vi "参数配置表.vi"() -> ()   [LabVIEW 2016, in "数据传输系统.lvlib"]
uses:
  <vilib>/Utility/miscctls.llb/LVPointTypeDef.ctl
  <vilib>/Utility/config.llb/NI_LVConfig.lvlib
  <vilib>/ptbypt/NI_PtbyPt.lvlib
panel:
  in  "加密传输":bool
  in  "数据库类型":enum16{"Access", "SQLite"}(ring)
  in  "应用环境":enum16{"STD", "GB212"}(ring)
  in  "屏蔽维护数据":bool
  in  "数据发送延时时间/s":i32
  in  "判断数据反馈":enum16{"非严格判断", "严格判断", "不判断"}(ring)
  in  "仪器参数发送":bool
  in  "地表水/污染源":bool
  in  "间隔时间/分钟":i32
  in  "数据发送通道":enum16{"TCP", "VISA"}(ring)
  in  "数据发送协议":enum16{"2005-212协议", "2017-212协议"}(ring)=enum."2017-212协议"
  in  "数据触发上传方式":enum16{"出数即刻发送", "间隔时间发送", "整点发送"}(ring)
  in  "数据组合发送":bool
  in  "日志、参数发送":bool
  in  "2011发送":bool
  in  "返回":bool
  out "配置表格":string[][](table)
  in  "参数数值":T1={"CODMn"=TRUE, "CODCr"=TRUE, "DO"=TRUE, "铜"=TRUE, "PH"=TRUE, "氨氮"=TRUE, "比电导率"=TRUE, "水温"=TRUE, "COD"=TRUE, "浊度"=TRUE, "总氮"=TRUE, "总磷"=TRUE, "叶绿素a"=TRUE, "藻密度"=TRUE, "水位"=TRUE, "流速"=TRUE, "瞬时流量"=TRUE, "累积流量"=TRUE, "亚硝氮"=TRUE, "硫化物"=TRUE, "ORP"=TRUE, "铅"=TRUE, "镉"=TRUE, "锌"=TRUE, "镍"=TRUE, "锰"=TRUE, "汞"=TRUE, "气温"=TRUE, "气压"=TRUE, "风速"=TRUE, "风向"=TRUE, "盐度"=TRUE, "磷酸盐"=TRUE, "硝氮"=TRUE, "氟化物"=TRUE}
  # "因子编码，单位配置，上传功能码，小时、质控数据上传触发方式"
  # "参数配置"
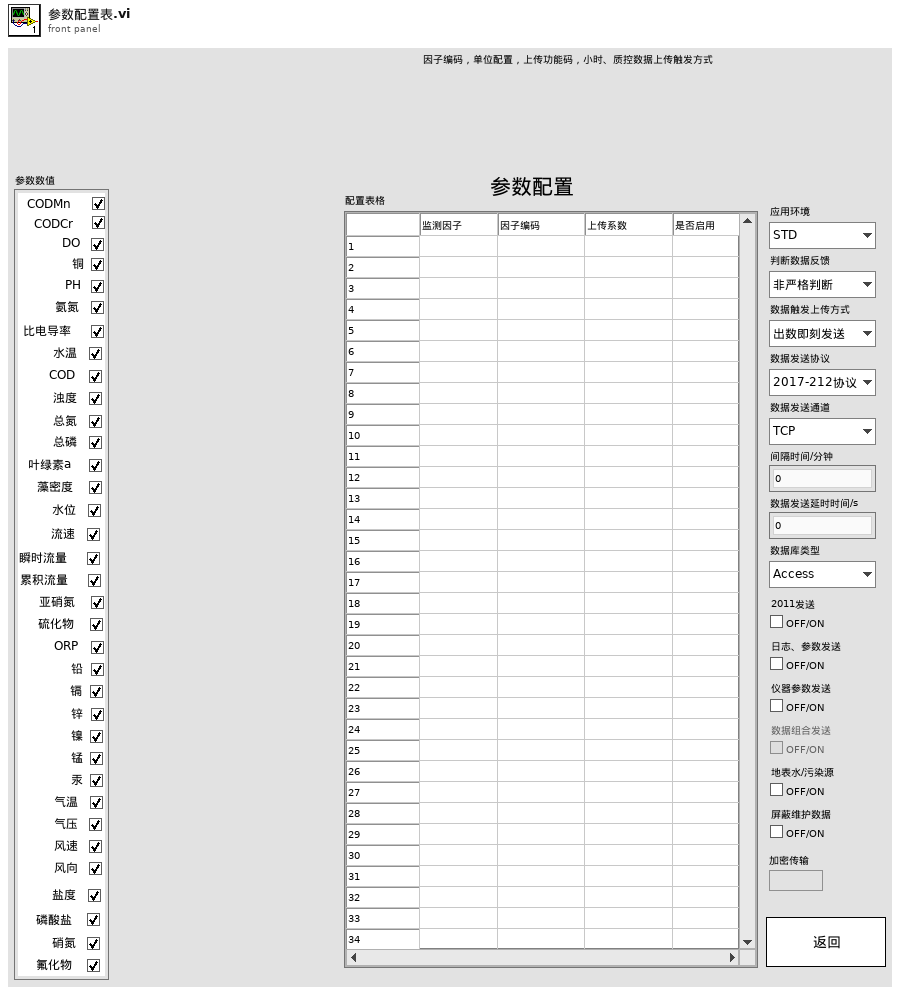
[diagram p1: front panel]
types:
  T1 = cluster{"CODMn":bool, "CODCr":bool, "DO":bool, "铜":bool, "PH":bool, "氨氮":bool, "比电导率":bool, "水温":bool, "COD":bool, "浊度":bool, "总氮":bool, "总磷":bool, "叶绿素a":bool, "藻密度":bool, "水位":bool, "流速":bool, "瞬时流量":bool, "累积流量":bool, "亚硝氮":bool, "硫化物":bool, "ORP":bool, "铅":bool, "镉":bool, "锌":bool, "镍":bool, "锰":bool, "汞":bool, "气温":bool, "气压":bool, "风速":bool, "风向":bool, "盐度":bool, "磷酸盐":bool, "硝氮":bool, "氟化物":bool}
  T2 = typedef "LVPointTypeDef.ctl" = cluster{"Horizontal":i16, "Vertical":i16}
  T3 = typedef "NI_LVConfig.lvlib/Config Data RefNum.ctl" = refnum<k1>
  T4 = cluster{"[0]":string, "[1]":string, "[2]":string, "[3]":string, "[4]":string, "[5]":string, "[6]":string, "[7]":string, "[8]":string, "[9]":string, "[10]":string, "[11]":string, "[12]":string, "[13]":string, "[14]":string, "[15]":string, "[16]":string, "[17]":string, "[18]":string, "[19]":string, "[20]":string, "[21]":string, "[22]":string, "[23]":string, "[24]":string, "[25]":string, "[26]":string, "[27]":string, "[28]":string, "[29]":string, "[30]":string, "[31]":string, "[32]":string, "[33]":string, "[34]":string}
  T5 = enum8{"Enabled", "Disabled", "Disabled and Grayed Out"}
  T6 = typedef "LVRowAndColumnTypeDef.ctl" = cluster{"Row":i32, "Column":i32}
  T7 = cluster{"[0]":string, "[1]":string, "[2]":string, "[3]":string, "[4]":string, "[5]":string, "[6]":string}
  T8 = cluster{"[0]":string, "[1]":string, "[2]":string, "[3]":string, "[4]":string, "[5]":string, "[6]":string, "[7]":string, "[8]":string, "[9]":string, "[10]":string, "[11]":string, "[12]":string}
  T9 = cluster{"[0]":string, "[1]":string, "[2]":string, "[3]":string, "[4]":string, "[5]":string, "[6]":string, "[7]":string, "[8]":string, "[9]":string, "[10]":string, "[11]":string, "[12]":string, "[13]":string}
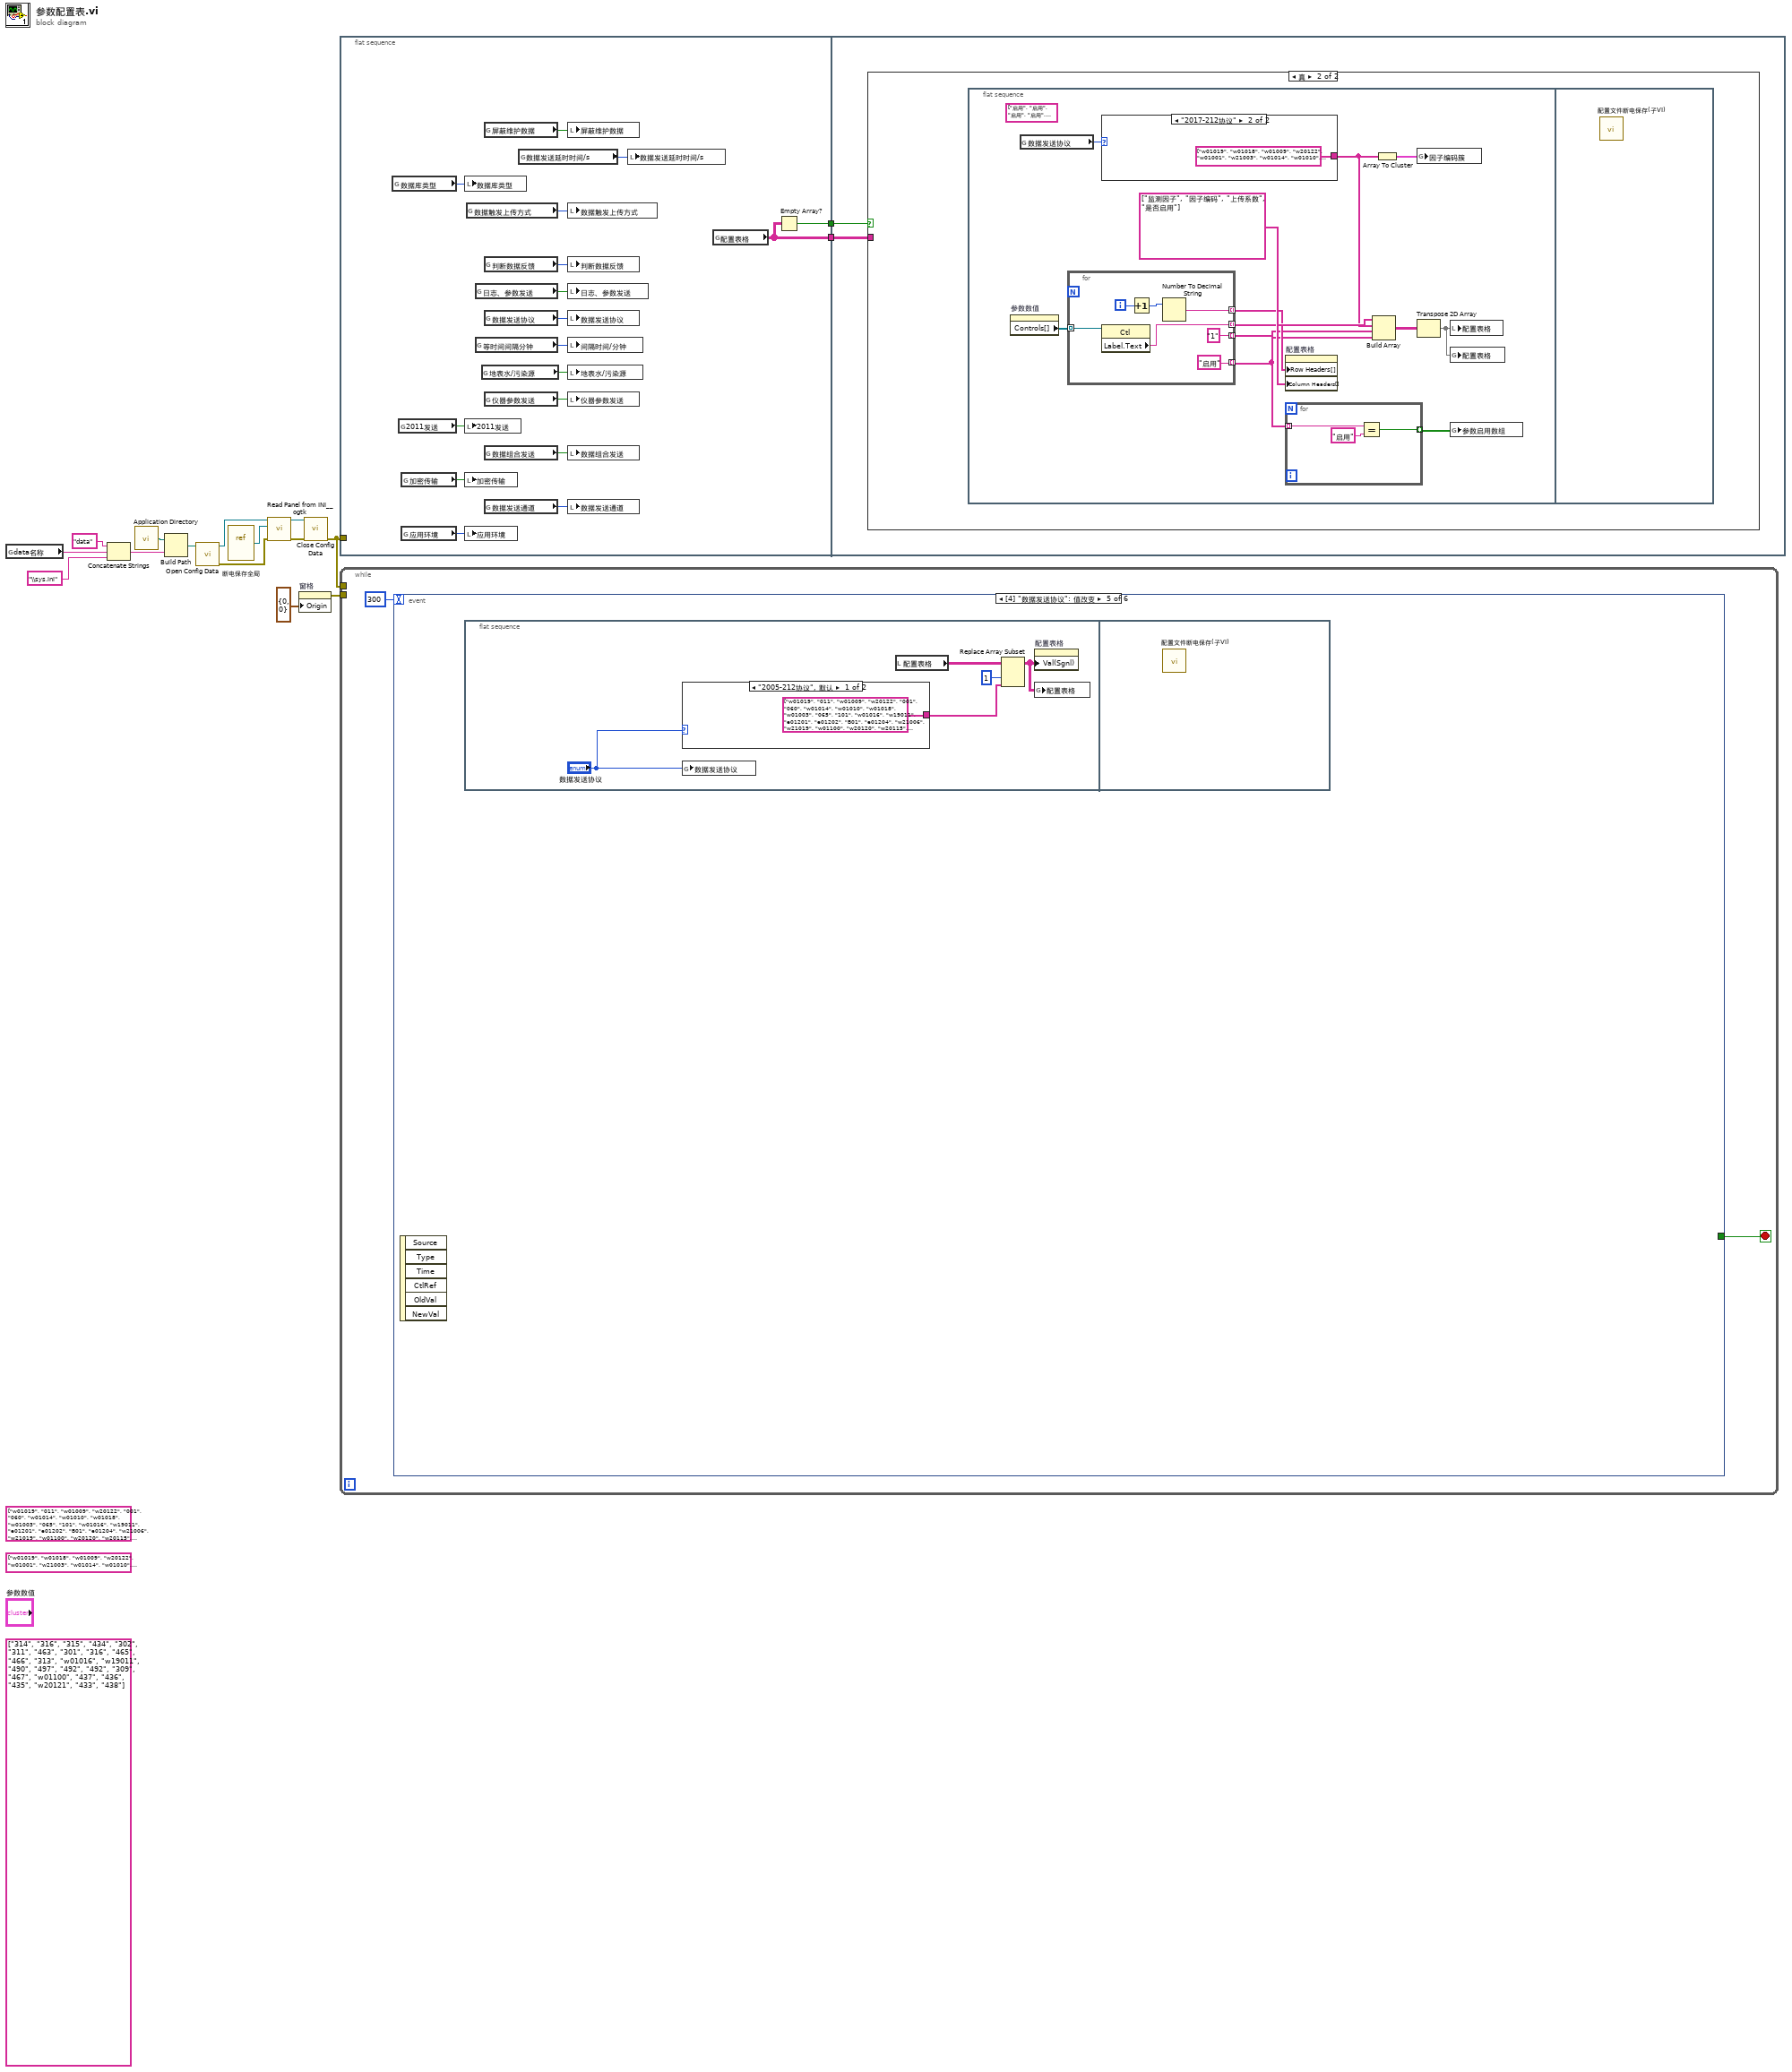
[diagram p0: block diagram]
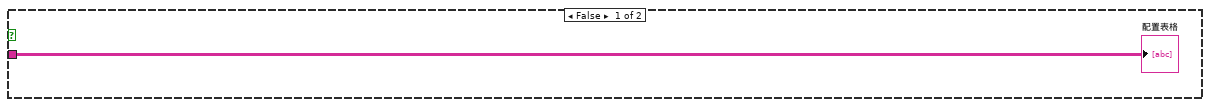
[diagram p2: hidden frame]
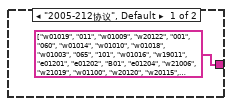
[diagram p3: hidden frame]
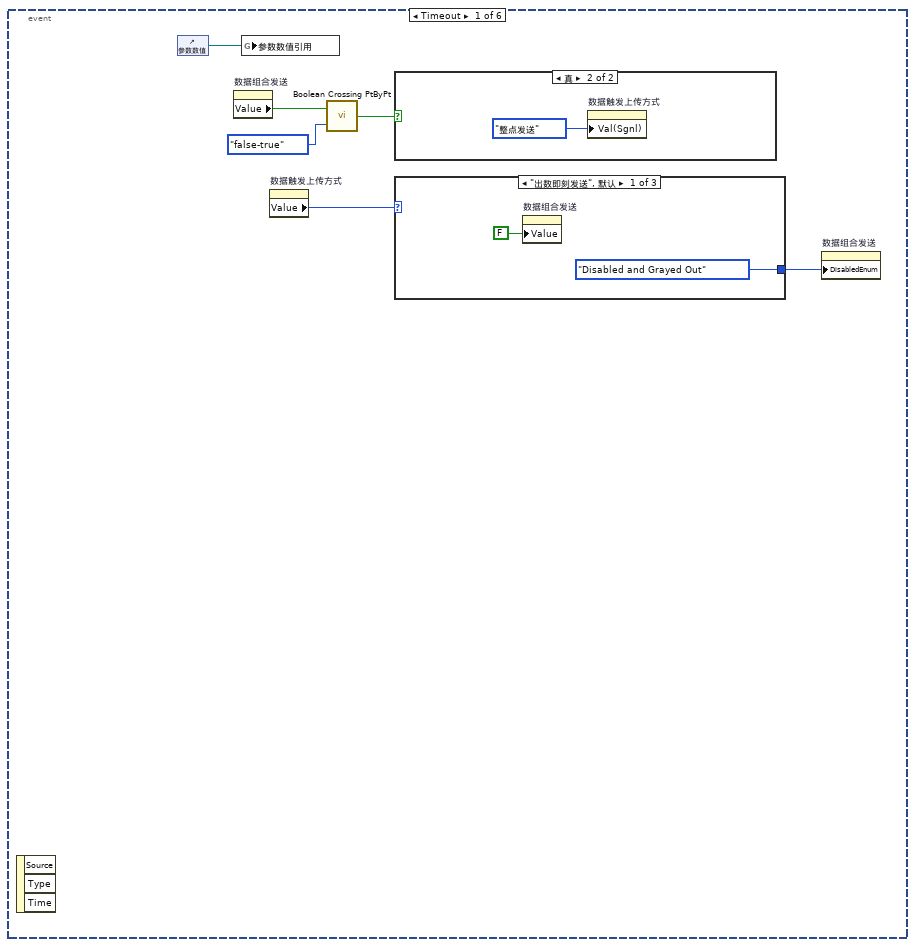
[diagram p4: hidden frame]
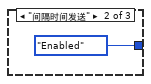
[diagram p6: hidden frame]
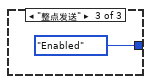
[diagram p7: hidden frame]
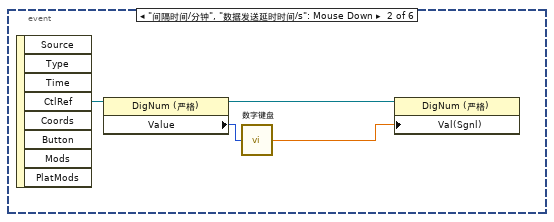
[diagram p8: hidden frame]
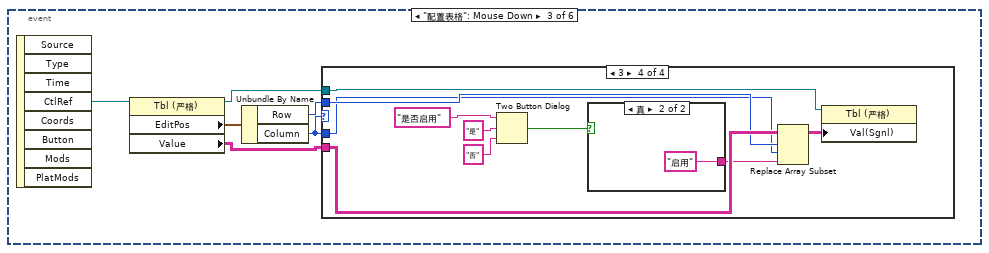
[diagram p9: hidden frame]
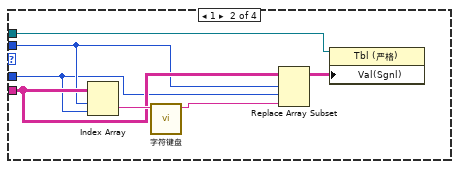
[diagram p11: hidden frame]
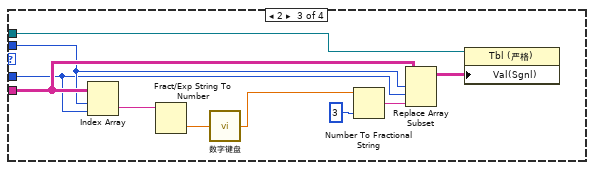
[diagram p12: hidden frame]
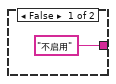
[diagram p13: hidden frame]
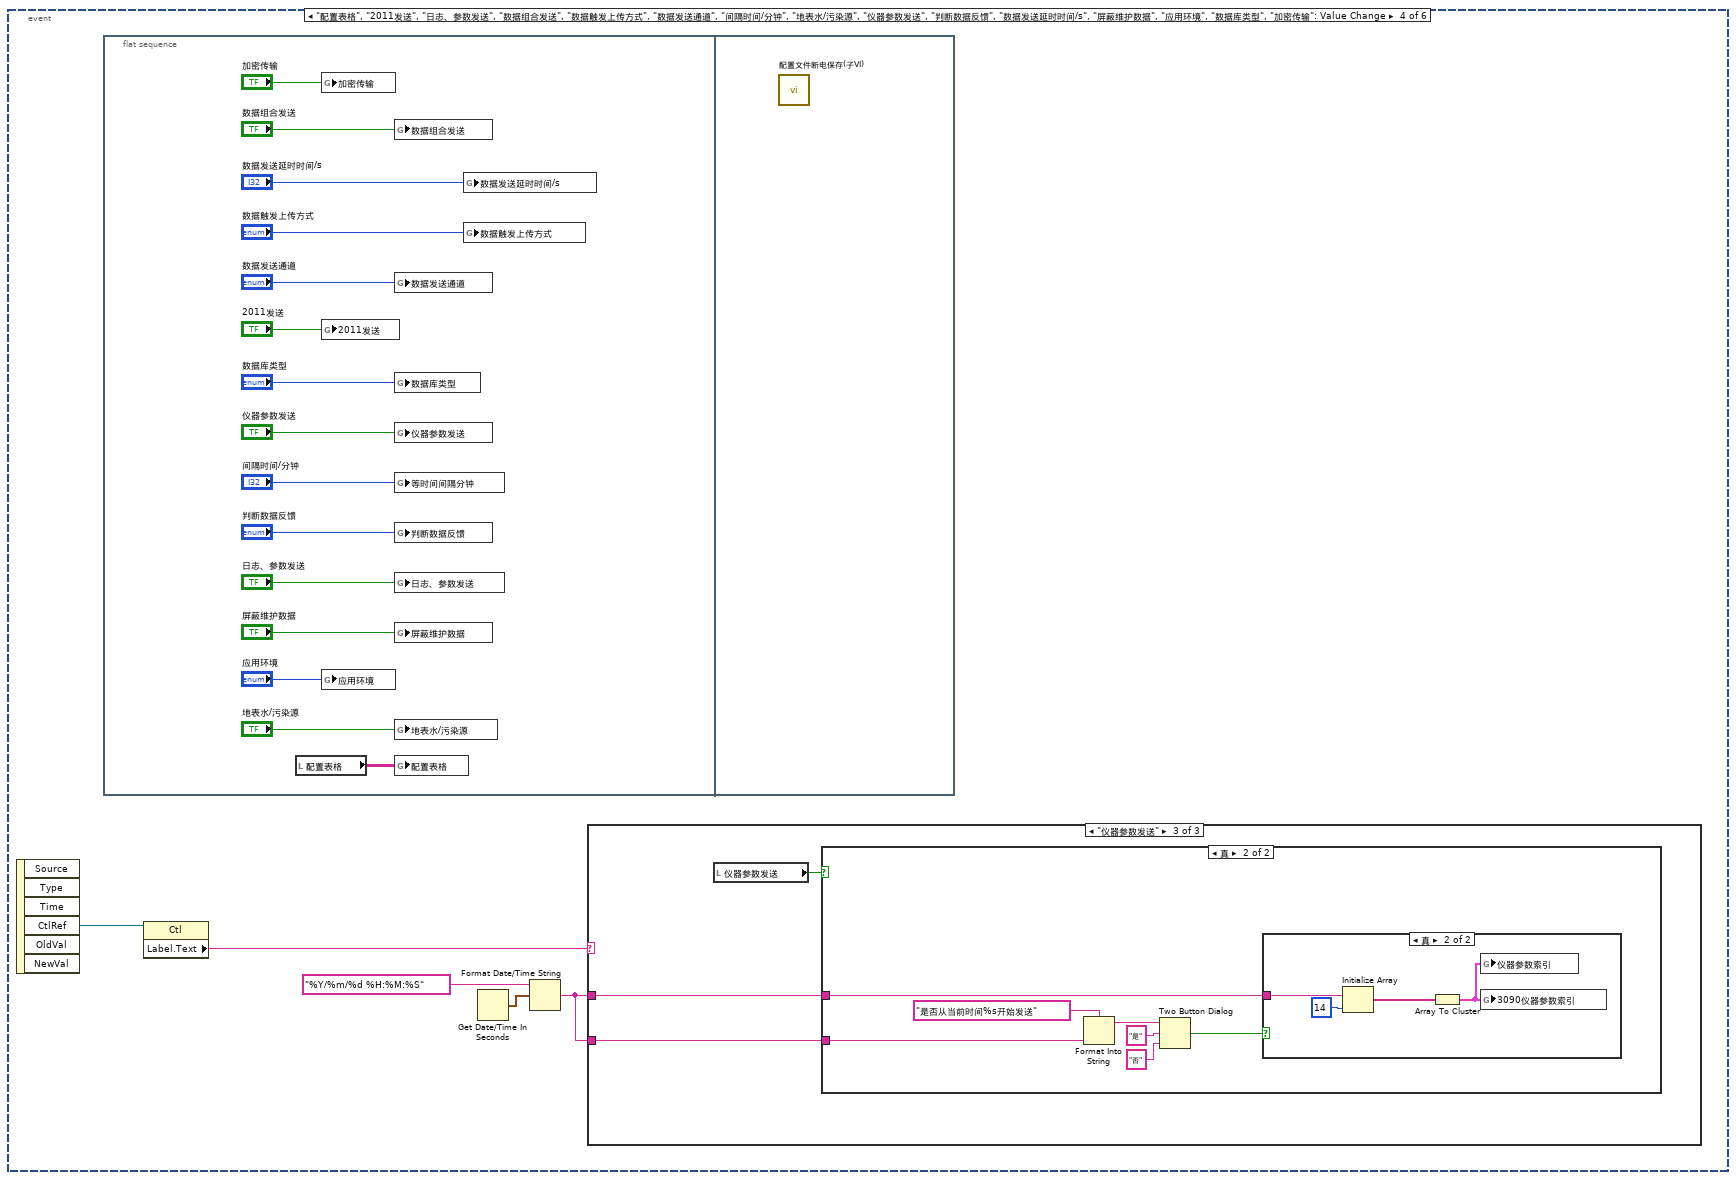
[diagram p14: hidden frame]
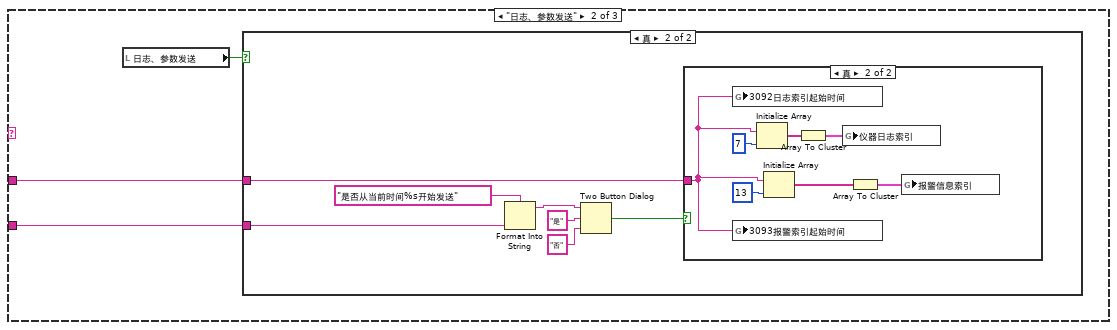
[diagram p16: hidden frame]
diagram:
  (unwired) string[] ["w01019", "011", "w01009", "w20122", "001", "060", "w01014", "w01010", "w01018", "w01003", "065", "101", "w01016", "w19011", "e01201", "e01202", "B01", "e01204", "w21006", "w21019", "w01100", "w20120", "w20115", "w20123", "w20121", "w20124", "w20111", "a01001", "a01006", "a01007", "a01008", "w01002", "w21015", "w21007", "w21017"]
  (unwired) string[] ["w01019", "w01018", "w01009", "w20122", "w01001", "w21003", "w01014", "w01010", "w01018", "w01003", "w21001", "w21011", "w01016", "w19011", "e01201", "e01202", "e01203", "e01204", "w21006", "w21019", "w01100", "w20120", "w20115", "w20123", "w20121", "w20124", "w20111", "a01001", "a01006", "a01007", "a01008", "w01002", "w21015", "w21007", "w21017"]
  (unwired) string[] ["314", "316", "315", "434", "302", "311", "463", "301", "316", "465", "466", "313", "w01016", "w19011", "490", "497", "492", "492", "309", "467", "w01100", "437", "436", "435", "w20121", "433", "438"]
  n1 = global read "断电保存全局.vi" "data名称"() -> (w3:string)
  n2 = Concatenate Strings("data" ("名称或相对路径"), w3, "\\sys.ini" ("名称或相对路径")) -> (w1:string)
  n3 = call <vilib>:"Application Directory.vi"() -> ("Application Directory"=w12:path)
  n4 = Build Path(base path=w12, name or relative path=w1) -> (appended path=w11:path)
  n5 = call <vilib>:"Open Config Data.vi"("configuration file path"=w11) -> ("error out"=w16:errorcluster, "refnum"=w15:T3)  [unwired: 8 in, 1 out]
  n6 = vi-ref "断电保存全局.vi"() -> (w14:refnum<vi>)
  n7 = call <userlib>:"Read Panel from INI__ogtk.vi"("error in (no error)"=w16, "VI ref"=w14, "refnum"=w15) -> ("error out"=w10:errorcluster, "refnum out"=w13:T3)  [unwired: 7 in]
  n8 = property on="窗格" class="Pane"("Origin"=T2 {"Horizontal"=0, "Vertical"=0} ("原点")) -> (error out=w8:errorcluster)  [unwired: 2 in, 1 out]
  n9 = call <vilib>:"Close Config Data.vi"("error in (no error)"=w10, "refnum"=w13) -> ("error out"=w9:errorcluster)  [unwired: 8 in, 1 out]
  n10 = flat-sequence {
    tunnel: w9 -> [_]
    tunnel: [w26] -> w6
    tunnel: [w25] -> w5
    tunnel: w6 -> [w35]
    tunnel: w5 -> [w34]
    frame #0 {
      n11 = global read "断电保存全局.vi" "数据库类型"() -> (w18:enum16{"Access", "SQLite"})
      n12 = global read "断电保存全局.vi" "2011发送"() -> (w33:bool)
      n13 = global read "断电保存全局.vi" "加密传输"() -> (w17:bool)
      n14 = global read "断电保存全局.vi" "应用环境"() -> (w19:enum16{"STD", "GB212"})
      n15 = local write "数据库类型"(w18) -> ()
      n16 = local write "2011发送"(w33) -> ()
      n17 = local write "加密传输"(w17) -> ()
      n18 = local write "应用环境"(w19) -> ()
      n19 = global read "断电保存全局.vi" "数据触发上传方式"() -> (w29:enum16{"出数即刻发送", "间隔时间发送", "整点发送"})
      n20 = global read "断电保存全局.vi" "日志、参数发送"() -> (w31:bool)
      n21 = global read "断电保存全局.vi" "等时间间隔分钟"() -> (w24:i32)
      n22 = global read "断电保存全局.vi" "地表水/污染源"() -> (w23:bool)
      n23 = global read "断电保存全局.vi" "屏蔽维护数据"() -> (w20:bool)
      n24 = global read "断电保存全局.vi" "判断数据反馈"() -> (w32:enum16{"非严格判断", "严格判断", "不判断"})
      n25 = global read "断电保存全局.vi" "数据发送协议"() -> (w27:enum16{"2005-212协议", "2017-212协议"})
      n26 = global read "断电保存全局.vi" "仪器参数发送"() -> (w22:bool)
      n27 = global read "断电保存全局.vi" "数据组合发送"() -> (w30:bool)
      n28 = global read "断电保存全局.vi" "数据发送通道"() -> (w28:enum16{"TCP", "VISA"})
      n29 = global read "断电保存全局.vi" "数据发送延时时间/s"() -> (w21:i32)
      n30 = local write "屏蔽维护数据"(w20) -> ()
      n31 = local write "数据触发上传方式"(w29) -> ()
      n32 = local write "判断数据反馈"(w32) -> ()
      n33 = local write "日志、参数发送"(w31) -> ()
      n34 = local write "数据发送协议"(w27) -> ()
      n35 = local write "间隔时间/分钟"(w24) -> ()
      n36 = local write "地表水/污染源"(w23) -> ()
      n37 = local write "仪器参数发送"(w22) -> ()
      n38 = local write "数据组合发送"(w30) -> ()
      n39 = local write "数据发送通道"(w28) -> ()
      n40 = local write "数据发送延时时间/s"(w21) -> ()
      n41 = global read "断电保存全局.vi" "配置表格"() -> (w25:string[][])
      n42 = Empty Array?(array=w25) -> (empty?=w26:bool)
    }
    frame #1 {
      n43 = case shown="真" w35 {
        tunnel: w34 -> [w36 _]
        frame False {
          "配置表格" <- w36
        }
        frame True {
          n44 = flat-sequence {
            frame #0 {
              (unwired) string[] ["启用", "启用", "启用", "启用", "启用", "启用", "启用", "启用", "启用", "启用", "启用", "启用", "启用", "启用", "启用", "启用", "启用", "启用", "启用", "启用", "启用", "启用", "启用", "启用", "启用", "启用", "启用"]
              n45 = property on="参数数值" class="Clust (严格)"() -> ("Controls[]"=w44:refnum<vi>[])  [unwired: 2 in, 2 out]
              n46 = global read "断电保存全局.vi" "数据发送协议"() -> (w42:enum16{"2005-212协议", "2017-212协议"})
              n47 = for {
                tunnel: w44 -> [w60] mode=indexing
                tunnel: [w59] -> w46 mode=indexing
                tunnel: [w57] -> w45 mode=indexing
                tunnel: ["1"] -> w39 mode=indexing
                tunnel: ["启用"] -> w37 mode=indexing
                i -> [w58]
                n48 = property class="Ctl"(reference=w60) -> ("Label.Text"=w59:string)  [unwired: 1 in, 2 out]
                n49 = Increment(x=w58) -> (x+1=w56:i32)
                n50 = Number To Decimal String(number=w56) -> (decimal integer string=w57:string)  [unwired: 1 in]
              }
              n51 = case shown="\"2017-212协议\"" w42 {
                tunnel: [string[] ["w01019", "011", "w01009", "w20122", "001", "060", "w01014", "w01010", "w01018", "w01003", "065", "101", "w01016", "w19011", "e01201", "e01202", "B01", "e01204", "w21006", "w21019", "w01100", "w20120", "w20115", "w20123", "w20121", "w20124", "w20111", "a01001", "a01006", "a01007", "a01008", "w01002", "w21015", "w21007", "w21017"] string[] ["w01019", "w01018", "w01009", "w20122", "w01001", "w21003", "w01014", "w01010", "w01018", "w01003", "w21001", "w21011", "w01016", "w19011", "e01201", "e01202", "e01203", "e01204", "w21006", "w21019", "w01100", "w20120", "w20115", "w20123", "w20121", "w20124", "w20111", "a01001", "a01006", "a01007", "a01008", "w01002", "w21015", "w21007", "w21017"]] -> w40
                frame "2005-212协议", Default {
                }
                frame "2017-212协议" {
                }
              }
              n52 = property on="配置表格" class="Tbl (严格)"("Row Headers[]"=w45, "Column Headers[]"=string[] ["监测因子", "因子编码", "上传系数", "是否启用"]) -> ()  [unwired: 2 in, 2 out]
              n53 = for {
                tunnel: w37 -> [w51] mode=indexing
                tunnel: [w49] -> w38 mode=indexing
                n54 = Equal?(x=w51, y="启用") -> (x = y?=w49:bool)
              }
              n55 = Build Array(w46, w40, w39, w37) -> (w48:string[][])
              n56 = Array To Cluster(array=w40) -> (cluster=w41:T4)
              n57 = global write "断电保存全局.vi" "因子编码簇"(w41) -> ()
              n58 = Transpose 2D Array(2D array=w48) -> (transposed array=w43:string[][])
              n59 = local write "配置表格"(w43) -> ()
              n60 = global write "断电保存全局.vi" "配置表格"(w43) -> ()
              n61 = global write "断电保存全局.vi" "参数启用数组"(w38) -> ()
            }
            frame #1 {
              n62 = call "配置文件断电保存(子VI).vi"() -> ()  [unwired: 12 in]
            }
          }
        }
      }
    }
  }
  n63 = while {
    tunnel: w9 -> [_]
    tunnel: w8 -> [_]
    stop <- w61 stop-if-true
    n64 = event shown="[4] \"数据发送协议\": 值改变" {
      selector: _ -> [_ _ _ _ _ _]
      dyn-events: _ -> [_ _ _ _ _ _]
      timeout: 300 -> [_ _ _ _ _ _]
      tunnel: [_ _ _ _ _ TRUE] -> w61
      event Timeout {
        n65 = event-data() -> ()  [unwired: 1 in, 3 out]
        n66 = control-ref of="参数数值"() -> (w63:refnum<vi>)
        n67 = property on="数据组合发送" class="Bool (严格)"() -> ("Value"=w66:bool)  [unwired: 2 in, 2 out]
        n68 = global write "断电保存全局.vi" "参数数值引用"(w63) -> ()
        n69 = property on="数据触发上传方式" class="Enum (严格)"() -> ("Value"=w68:enum16{"出数即刻发送", "间隔时间发送", "整点发送"})  [unwired: 2 in, 2 out]
        n70 = call <vilib>:"Boolean Crossing PtByPt.vi"("direction"=enum16{"either", "false-true", "true-false"}."false-true", "input"=w66) -> ("crossing"=w64:bool)  [unwired: 1 in]
        n71 = case shown="真" w64 {
          frame False {
          }
          frame True {
            n72 = property on="数据触发上传方式" class="Enum (严格)"("Val(Sgnl)"=enum16{"出数即刻发送", "间隔时间发送", "整点发送"}."整点发送" ("值(信号)")) -> ()  [unwired: 2 in, 2 out]
          }
        }
        n73 = case shown="\"出数即刻发送\", 默认" w68 {
          tunnel: [T5."Disabled and Grayed Out" ("禁用") T5."Enabled" ("禁用") T5."Enabled" ("禁用")] -> w67
          frame "出数即刻发送", Default {
            n74 = property on="数据组合发送" class="Bool (严格)"("Value"=FALSE ("值(信号)")) -> ()  [unwired: 2 in, 2 out]
          }
          frame "间隔时间发送" {
          }
          frame "整点发送" {
          }
        }
        n75 = property on="数据组合发送" class="Bool (严格)"("DisabledEnum"=w67) -> ()  [unwired: 2 in, 2 out]
      }
      event "间隔时间/分钟", "数据发送延时时间/s": Mouse Down {
        n76 = event-data() -> ("CtlRef"=w77:refnum<vi>)  [unwired: 1 in, 7 out]
        n77 = property class="DigNum (严格)"(reference=w77) -> (reference out=w75:refnum<vi>, "Value"=w76:i32)  [unwired: 1 in, 1 out]
        n78 = call "数字键盘.vi"("OldNumber"=w76) -> ("NewNumber"=w74:sgl)
        n79 = property class="DigNum (严格)"(reference=w75, "Val(Sgnl)"=w74) -> ()  [unwired: 1 in, 2 out]
      }
      event "配置表格": Mouse Down {
        n80 = event-data() -> ("CtlRef"=w83:refnum<vi>)  [unwired: 1 in, 7 out]
        n81 = property class="Tbl (严格)"(reference=w83) -> (reference out=w79:refnum<vi>, "EditPos"=w82:T6, "Value"=w81:string[][])  [unwired: 1 in, 1 out]
        n82 = Unbundle By Name(w82) -> ("Row"=w80:i32, "Column"=w78:i32)
        n83 = case shown="3" w78 {
          tunnel: w81 -> [_ w89 w100 w104]
          tunnel: w80 -> [_ w88 w99 w103]
          tunnel: w78 -> [_ w87 w98 w102]
          tunnel: w79 -> [_ w85 w97 w105]
          frame 0, Default {
          }
          frame 1 {
            n84 = Index Array(array=w89, index (row)=w88, index (col)=w87) -> (element=w90:string)
            n85 = call "字符键盘.vi"("原值"=w90) -> ("x+y"=w86:string)  [unwired: 10 in]
            n86 = Replace Array Subset(array=w89, new element=w86, index (row)=w88, index (col)=w87) -> (w84:string[][])
            n87 = property class="Tbl (严格)"(reference=w85, "Val(Sgnl)"=w84) -> ()  [unwired: 1 in, 2 out]
          }
          frame 2 {
            n88 = Index Array(array=w100, index (row)=w99, index (col)=w98) -> (element=w95:string)
            n89 = Fract/Exp String To Number(string=w95) -> (number=w94:dbl)  [unwired: 3 in, 1 out]
            n90 = call "数字键盘.vi"("OldNumber"=w94) -> ("NewNumber"=w93:sgl)
            n91 = Number To Fractional String(number=w93, precision (6)=i16 3 ("精度(6)")) -> (F-format string=w92:string)  [unwired: 2 in]
            n92 = Replace Array Subset(array=w100, new element=w92, index (row)=w99, index (col)=w98) -> (w96:string[][])
            n93 = property class="Tbl (严格)"(reference=w97, "Val(Sgnl)"=w96) -> ()  [unwired: 1 in, 2 out]
          }
          frame 3 {
            n94 = Two Button Dialog(message="是否启用" ("消息"), 1:"否" ("F按钮名称（“取消”）"), 2:"是" ("T按钮名称（“确定”）")) -> (T button?=w107:bool)
            n95 = case shown="真" w107 {
              tunnel: ["不启用" "启用"] -> w101
              frame False {
              }
              frame True {
              }
            }
            n96 = Replace Array Subset(array=w104, new element=w101, index (row)=w103, index (col)=w102) -> (w106:string[][])
            n97 = property class="Tbl (严格)"(reference=w105, "Val(Sgnl)"=w106) -> ()  [unwired: 1 in, 2 out]
          }
        }
      }
      event "配置表格", "2011发送", "日志、参数发送", "数据组合发送", "数据触发上传方式", "数据发送通道", "间隔时间/分钟", "地表水/污染源", "仪器参数发送", "判断数据反馈", "数据发送延时时间/s", "屏蔽维护数据", "应用环境", "数据库类型", "加密传输": Value Change {
        n98 = event-data() -> ("CtlRef"=w117:refnum<vi>)  [unwired: 1 in, 5 out]
        n99 = flat-sequence {
          frame #0 {
            n100 = local read "配置表格"() -> (w163:string[][])
            n101 = global write "断电保存全局.vi" "加密传输"("加密传输") -> ()
            n102 = global write "断电保存全局.vi" "2011发送"("2011发送") -> ()
            n103 = global write "断电保存全局.vi" "应用环境"("应用环境") -> ()
            n104 = global write "断电保存全局.vi" "数据组合发送"("数据组合发送") -> ()
            n105 = global write "断电保存全局.vi" "数据发送通道"("数据发送通道") -> ()
            n106 = global write "断电保存全局.vi" "数据库类型"("数据库类型") -> ()
            n107 = global write "断电保存全局.vi" "仪器参数发送"("仪器参数发送") -> ()
            n108 = global write "断电保存全局.vi" "等时间间隔分钟"("间隔时间/分钟") -> ()
            n109 = global write "断电保存全局.vi" "判断数据反馈"("判断数据反馈") -> ()
            n110 = global write "断电保存全局.vi" "日志、参数发送"("日志、参数发送") -> ()
            n111 = global write "断电保存全局.vi" "屏蔽维护数据"("屏蔽维护数据") -> ()
            n112 = global write "断电保存全局.vi" "地表水/污染源"("地表水/污染源") -> ()
            n113 = global write "断电保存全局.vi" "配置表格"(w163) -> ()
            n114 = global write "断电保存全局.vi" "数据发送延时时间/s"("数据发送延时时间/s") -> ()
            n115 = global write "断电保存全局.vi" "数据触发上传方式"("数据触发上传方式") -> ()
          }
          frame #1 {
            n116 = call "配置文件断电保存(子VI).vi"() -> ()  [unwired: 12 in]
          }
        }
        n117 = property class="Ctl"(reference=w117) -> ("Label.Text"=w116:string)  [unwired: 1 in, 2 out]
        n118 = Get Date/Time In Seconds() -> (seconds since 1Jan1904=w115:timestamp)
        n119 = Format Date/Time String(time format string (%c)="%Y/%m/%d %H:%M:%S" ("时间格式字符串(%c)"), seconds (now)=w115) -> (date/time string=w113:string)  [unwired: 1 in]
        n120 = case shown="\"仪器参数发送\"" w116 {
          tunnel: w113 -> [_ w119 w136]
          tunnel: w113 -> [_ w118 w135]
          frame "假", Default {
          }
          frame "日志、参数发送" {
            n121 = local read "日志、参数发送"() -> (w120:bool)
            n122 = case shown="真" w120 {
              tunnel: w119 -> [_ w124]
              tunnel: w118 -> [_ w122]
              frame False {
              }
              frame True {
                n123 = Format Into String(format string="是否从当前时间%s开始发送" ("消息"), w122) -> (resulting string=w121:string)  [unwired: 2 in, 1 out]
                n124 = Two Button Dialog(message=w121, 1:"否" ("F按钮名称（“取消”）"), 2:"是" ("T按钮名称（“确定”）")) -> (T button?=w125:bool)
                n125 = case shown="真" w125 {
                  tunnel: w124 -> [_ w128]
                  frame False {
                  }
                  frame True {
                    n126 = global write "全局 时间2.vi" "3092日志索引起始时间"(w128) -> ()
                    n127 = global write "全局 时间2.vi" "3093报警索引起始时间"(w128) -> ()
                    n128 = Initialize Array(w128, 7 ("维数大小")) -> (w129:string[])
                    n129 = Initialize Array(w128, 13 ("维数大小")) -> (w132:string[])
                    n130 = Array To Cluster(array=w129) -> (cluster=w130:T7)
                    n131 = global write "全局 时间2.vi" "仪器日志索引"(w130) -> ()
                    n132 = Array To Cluster(array=w132) -> (cluster=w131:T8)
                    n133 = global write "全局 时间2.vi" "报警信息索引"(w131) -> ()
                  }
                }
              }
            }
          }
          frame "仪器参数发送" {
            n134 = local read "仪器参数发送"() -> (w137:bool)
            n135 = case shown="真" w137 {
              tunnel: w136 -> [_ w141]
              tunnel: w135 -> [_ w139]
              frame False {
              }
              frame True {
                n136 = Format Into String(format string="是否从当前时间%s开始发送" ("消息"), w139) -> (resulting string=w138:string)  [unwired: 2 in, 1 out]
                n137 = Two Button Dialog(message=w138, 1:"否" ("F按钮名称（“取消”）"), 2:"是" ("T按钮名称（“确定”）")) -> (T button?=w142:bool)
                n138 = case shown="真" w142 {
                  tunnel: w141 -> [_ w146]
                  frame False {
                  }
                  frame True {
                    n139 = Initialize Array(w146, 14 ("维数大小")) -> (w148:string[])
                    n140 = Array To Cluster(array=w148) -> (cluster=w145:T9)
                    n141 = global write "全局 时间2.vi" "仪器参数索引"(w145) -> ()
                    n142 = global write "全局 时间2.vi" "3090仪器参数索引"(w145) -> ()
                  }
                }
              }
            }
          }
        }
      }
      event "数据发送协议": Value Change {
        n143 = event-data() -> ()  [unwired: 1 in, 6 out]
        n144 = flat-sequence {
          frame #0 {
            n145 = case shown="\"2005-212协议\", 默认" "数据发送协议" {
              tunnel: [string[] ["w01019", "011", "w01009", "w20122", "001", "060", "w01014", "w01010", "w01018", "w01003", "065", "101", "w01016", "w19011", "e01201", "e01202", "B01", "e01204", "w21006", "w21019", "w01100", "w20120", "w20115", "w20123", "w20121", "w20124", "w20111", "a01001", "a01006", "a01007", "a01008", "w01002", "w21015", "w21007", "w21017"] string[] ["w01019", "w01018", "w01009", "w20122", "w01001", "w21003", "w01014", "w01010", "w01018", "w01003", "w21001", "w21011", "w01016", "w19011", "e01201", "e01202", "e01203", "e01204", "w21006", "w21019", "w01100", "w20120", "w20115", "w20123", "w20121", "w20124", "w20111", "a01001", "a01006", "a01007", "a01008", "w01002", "w21015", "w21007", "w21017"]] -> w166
              frame "2005-212协议", Default {
              }
              frame "2017-212协议" {
              }
            }
            n146 = global write "断电保存全局.vi" "数据发送协议"("数据发送协议") -> ()
            n147 = local read "配置表格"() -> (w167:string[][])
            n148 = Replace Array Subset(array=w167, new element=w166, index (col)=1 ("禁用的索引 (列)")) -> (w164:string[][])  [unwired: 1 in]
            n149 = property on="配置表格" class="Tbl (严格)"("Val(Sgnl)"=w164) -> ()  [unwired: 2 in, 2 out]
            n150 = global write "断电保存全局.vi" "配置表格"(w164) -> ()
          }
          frame #1 {
            n151 = call "配置文件断电保存(子VI).vi"() -> ()  [unwired: 12 in]
          }
        }
      }
      event "返回": Value Change; Panel Close {
        n152 = event-data() -> ()  [unwired: 1 in, 3 out]
      }
    }
  }
